vi "ttm_aecontrol_poller.vi"() -> ()   [LabVIEW 2011]
doc: "This is the sample data playback waveform and data logging example program. Sample data points are generated using MX Sample Data Array Generator.vi. You will need to replace this VI with your own code. New sample data is sent to the controller each time a status message is recieved from the controller that the next random buffer is running.\nThis program also shows you how to use Active X events. These are used to notify the program when a data buffer is ready for collection and when to load a new buffer of sample data points. Two separate event queues are used: one for data logging and the other for general status, such as when a sample data point buffer can be sent to the controller. Each event handler must run in parallel loops as execution passes to MX Handle Status Change Event.vi and MX Handle Data Ready Event.vi and will not come out of them until an event is received from the console program. When modifiying this example for your own use you may want to setup a third loop to be doing other processing, or you could add code to manipulate the data buffer in the data monitoring loop."
panel:
  out "Number of points":i32=1000
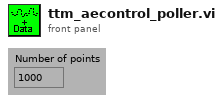
[diagram p1: front panel]
types:
  T1 = cluster{"Data Sample Format (0)":i8, "Loop code (2)":i8, "Target Amplitude (32767)":i16, "Playback rate":dbl, "Playback Scale":dbl[], "Envelope Ramp Rate":dbl, "Filter Order (0)":i8, "Filter Type (0)":i8, "Filter Bandwidth":dbl}
  T2 = cluster{"Name":string, "Type":i32, "SI Full Scale":dbl, "Full Scale":dbl, "Units String":string, "Display Format":string, "Gauge Length":dbl}[][]
  T3 = cluster{"Device ID":i32, "Device Name":string, "Device Type":i32}[]
  T4 = cluster{"Axis Information Out[0]":cluster{"Device ID":i32, "Device Name":string, "Device Type":i32}, "Axis Information Out[1]":cluster{"Device ID":i32, "Device Name":string, "Device Type":i32}, "Axis Information Out[2]":cluster{"Device ID":i32, "Device Name":string, "Device Type":i32}, "Axis Information Out[3]":cluster{"Device ID":i32, "Device Name":string, "Device Type":i32}, "Axis Information Out[4]":cluster{"Device ID":i32, "Device Name":string, "Device Type":i32}, "Axis Information Out[5]":cluster{"Device ID":i32, "Device Name":string, "Device Type":i32}, "Axis Information Out[6]":cluster{"Device ID":i32, "Device Name":string, "Device Type":i32}, "Axis Information Out[7]":cluster{"Device ID":i32, "Device Name":string, "Device Type":i32}, "Axis Information Out[8]":cluster{"Device ID":i32, "Device Name":string, "Device Type":i32}}
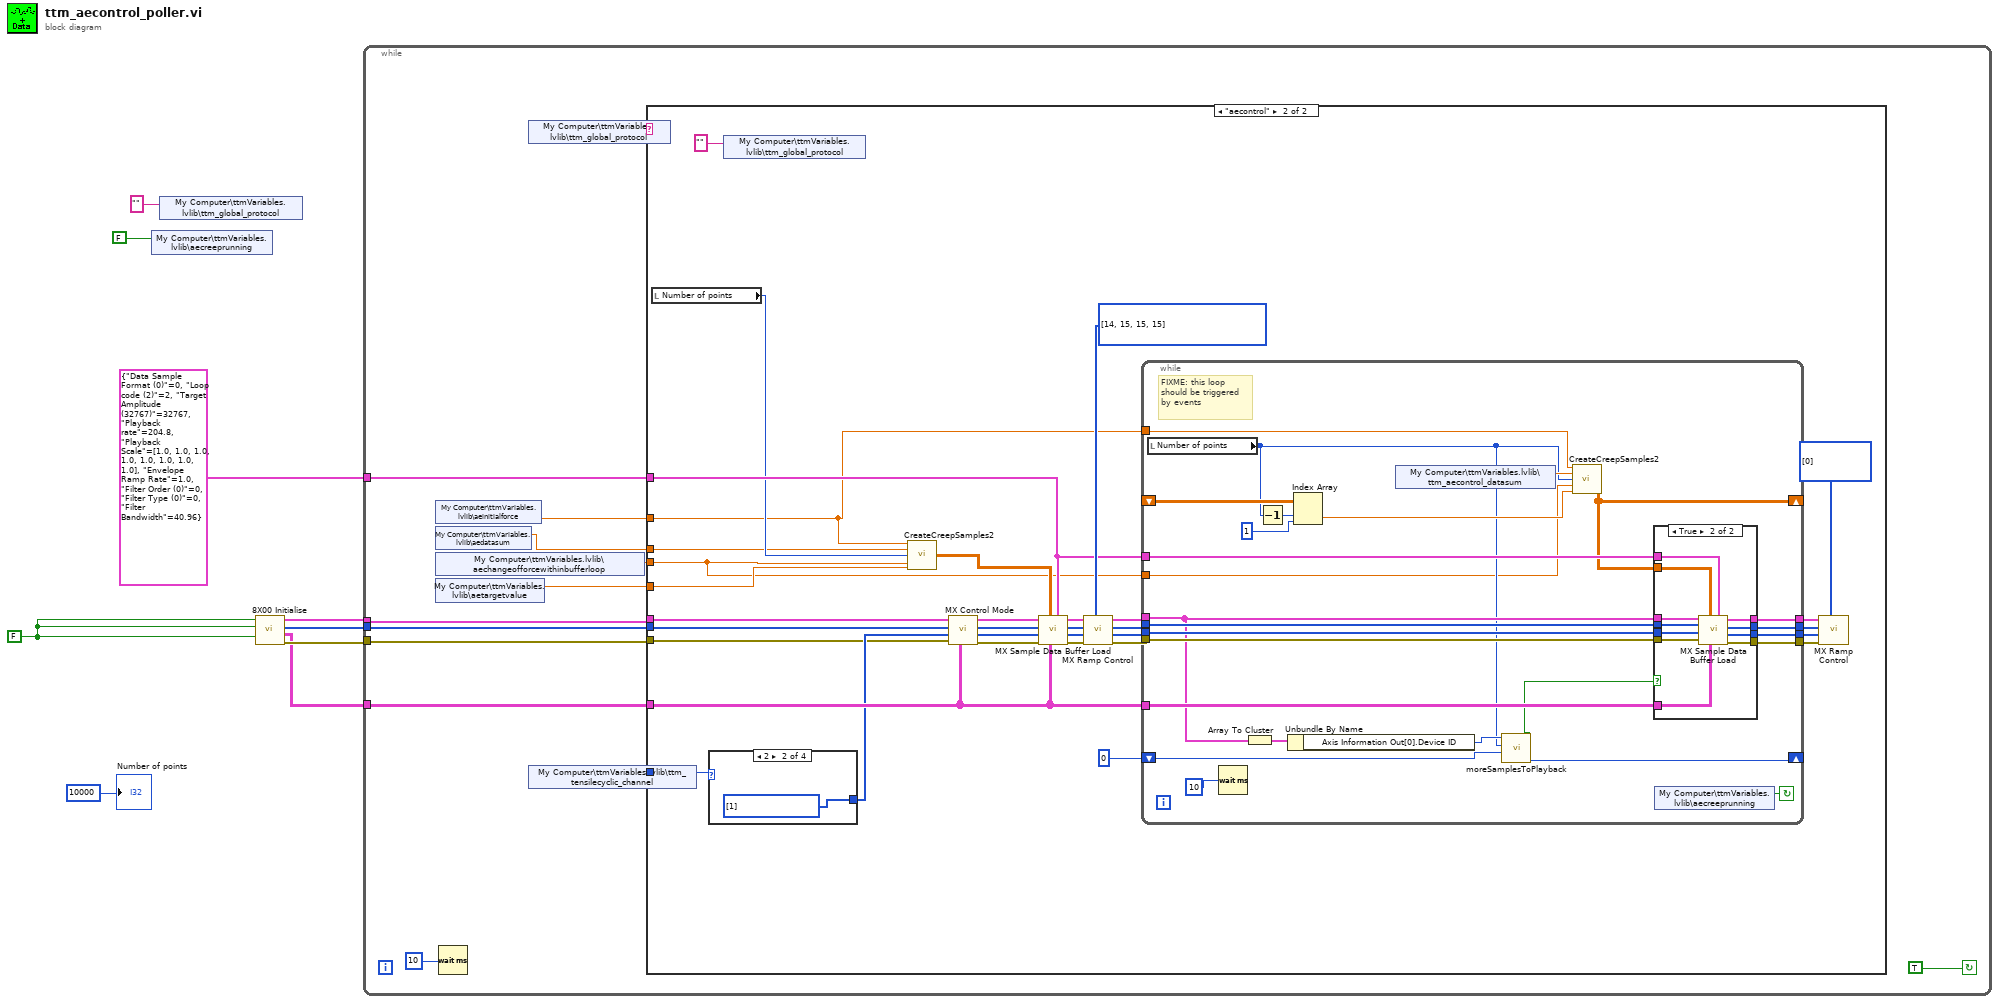
[diagram p0: block diagram]
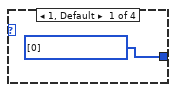
[diagram p3: hidden frame]
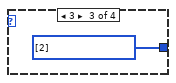
[diagram p4: hidden frame]
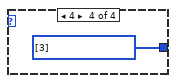
[diagram p5: hidden frame]
diagram:
  w6 = FALSE ("Reset")
  n1 = shared-variable "My Computer\\ttmVariables.lvlib\\aecreeprunning"(FALSE ("startCreep")) -> ()  [unwired: 1 in, 1 out]
  n2 = shared-variable "My Computer\\ttmVariables.lvlib\\ttm_global_protocol"("" ("protocol")) -> ()  [unwired: 1 in, 1 out]
  n3 = call "8X00 Initialise.vi"("Reset?"=w6, "Create DVM? (T)"=w6, "Create Console? (T)"=w6) -> ("error out"=w9:errorcluster, "Channel Data"=w8:T2, "Axis Selector"=w5:i32[], "Axis Information"=w7:T3)  [unwired: 1 in]
  n4 = while {
    tunnel: w8 -> [w22]
    tunnel: w7 -> [w18]
    tunnel: w9 -> [w16]
    tunnel: w5 -> [w17]
    tunnel: T1 {"Data Sample Format (0)"=0, "Loop code (2)"=2, "Target Amplitude (32767)"=32767, "Playback rate"=204.8, "Playback Scale"=[1.0, 1.0, 1.0, 1.0, 1.0, 1.0, 1.0, 1.0], "Envelope Ramp Rate"=1.0, "Filter Order (0)"=0, "Filter Type (0)"=0, "Filter Bandwidth"=40.96} ("Sample Data Playback Definition") -> [w14]
    stop <- TRUE continue-if-true
    n5 = shared-variable "My Computer\\ttmVariables.lvlib\\aeinitialforce"() -> (w12:dbl)  [unwired: 1 in, 1 out]
    n6 = shared-variable "My Computer\\ttmVariables.lvlib\\aedatasum"() -> (w13:dbl)  [unwired: 1 in, 1 out]
    n7 = shared-variable "My Computer\\ttmVariables.lvlib\\aechangeofforcewithinbufferloop"() -> (w11:dbl)  [unwired: 1 in, 1 out]
    n8 = shared-variable "My Computer\\ttmVariables.lvlib\\aetargetvalue"() -> (w19:dbl)  [unwired: 1 in, 1 out]
    n9 = Wait (ms)(milliseconds to wait=u32 10) -> ()  [unwired: 1 out]
    n10 = shared-variable "My Computer\\ttmVariables.lvlib\\ttm_global_protocol"() -> (w10:string)  [unwired: 1 in, 1 out]
    n11 = shared-variable "My Computer\\ttmVariables.lvlib\\ttm_tensilecyclic_channel"() -> (w15:i32)  [unwired: 1 in, 1 out]
    n12 = case shown="\"aecontrol\"" w10 {
      tunnel: w22 -> [_ w40]
      tunnel: w19 -> [_ w28]
      tunnel: w18 -> [_ w35]
      tunnel: w17 -> [_ w34]
      tunnel: w16 -> [_ w32]
      tunnel: w15 -> [_ w46]
      tunnel: w14 -> [_ w31]
      tunnel: w13 -> [_ w27]
      tunnel: w12 -> [_ w25]
      tunnel: w11 -> [_ w24]
      frame "False", Default {
      }
      frame "aecontrol" {
        w41 = u16[] [0] items=["Stop", "Start or continue", "Hold", "Continue", "Return ramp to set level at fixed rate", "Reserved", "Reserved", "Start Random without demand hold", "Start Random with demand hold", "Prepare Random Start without demand hold", "Prepare Random Start with demand hold", "Unslave", "Reserved", "Reserved", "Start Sample Data Playback or Resume", "Prepare for Start of Sample Data", "Reserved", "Reserved", "Resume Playback", "Start an electromechanical frame return"] ("Ramp Control")
        w51 = u16[] [14, 15, 15, 15] items=["Stop", "Start or continue", "Hold", "Continue", "Return ramp to set level at fixed rate", "Reserved", "Reserved", "Start Random without demand hold", "Start Random with demand hold", "Prepare Random Start without demand hold", "Prepare Random Start with demand hold", "Unslave", "Reserved", "Reserved", "Start Sample Data Playback or Resume", "Prepare for Start of Sample Data", "Reserved", "Reserved", "Resume Playback"] ("Ramp Control")
        n13 = local read "Number of points"() -> (w29:i32)
        n14 = case shown="2" w46 {
          tunnel: [w56 w57 w58 w59] -> w33
          frame 1, Default {
            w56 = u16[] [0] items=["Channel 1", "Channel 2", "Channel 3", "Channel 4"] ("Choose channel to apply\nthe setpoint")
          }
          frame 2 {
            w57 = u16[] [1] items=["Channel 1", "Channel 2", "Channel 3", "Channel 4"] ("Choose channel to apply\nthe setpoint")
          }
          frame 3 {
            w58 = u16[] [2] items=["Channel 1", "Channel 2", "Channel 3", "Channel 4"] ("Choose channel to apply\nthe setpoint")
          }
          frame 4 {
            w59 = u16[] [3] items=["Channel 1", "Channel 2", "Channel 3", "Channel 4"] ("Choose channel to apply\nthe setpoint")
          }
        }
        n15 = shared-variable "My Computer\\ttmVariables.lvlib\\ttm_global_protocol"("" ("protocol")) -> ()  [unwired: 1 in, 1 out]
        n16 = call "CreateCreepSamples2.vi"("setValueForAESum"=w25, "AEdataSum"=w27, "outputLength"=w29, "changeOfForceWithinBufferLoop"=w24, "initialOrPreviousForce"=w28) -> ("output array"=w30:dbl[][])  [unwired: 10 in]
        n17 = call "MX Control Mode.vi"("Channel Data"=w40, "error in (no error)"=w32, "Control Modes"=w33, "Axis Selector"=w34, "Axis Information"=w35) -> ("error out"=w36:errorcluster, "Control Modes out"=w37:u16[], "Axis Selector out"=w38:i32[], "Axis Information out"=w39:T3)  [unwired: 1 in]
        n18 = call "MX Sample Data Buffer Load.vi"("Sample Data Playback Definition"=w31, "Channel Data"=w40, "Sample Data"=w30, "error in (no error)"=w36, "Channels In"=w37, "Axis Selector In"=w38, "Axis Information In"=w39) -> ("error out"=w53:errorcluster, "Channels Out"=w52:u16[], "Axis Selector Out"=w54:i32[], "Axis Information Out"=w55:T3)  [unwired: 1 in]
        n19 = call "MX Ramp Control.vi"("Ramp Control"=w51, "error in (no error)"=w53, "Channels In"=w52, "Axis Selector In"=w54, "Axis Information In"=w55) -> ("error out"=w48:errorcluster, "Channels Out"=w50:u16[], "Axis Selector Out"=w49:i32[], "Axis Information Out"=w47:T3)  [unwired: 2 in]
        n20 = while {
          tunnel: w47 -> [w74]
          tunnel: w49 -> [w85]
          tunnel: w50 -> [w78]
          tunnel: w48 -> [w84]
          tunnel: [w75] -> w45
          tunnel: [w83] -> w44
          tunnel: [w82] -> w43
          tunnel: [w81] -> w42
          tunnel: w31 -> [w73]
          tunnel: w40 -> [w80]
          shift-right: [w69] -> _
          shift-left: _ -> [w72]
          shift-right: [w63] -> _
          shift-left: 0 -> [w62]
          tunnel: w25 -> [w61]
          tunnel: w24 -> [w60]
          stop <- w79 continue-if-true
          # "FIXME: this loop \nshould be triggered \nby events"
          n21 = local read "Number of points"() -> (w64:i32)
          n22 = Wait (ms)(milliseconds to wait=u32 10) -> ()  [unwired: 1 out]
          n23 = Array To Cluster(array=w74) -> (cluster=w76:T4)
          n24 = Decrement(x=w64) -> (x-1=w70:i32)
          n25 = Unbundle By Name(w76) -> ("Axis Information Out[0].Device ID"=w65:i32)
          n26 = Index Array(array=w72, index (row)=w70, index (col)=1) -> (element=w68:dbl)
          n27 = shared-variable "My Computer\\ttmVariables.lvlib\\ttm_aecontrol_datasum"() -> (w67:dbl)  [unwired: 1 in, 1 out]
          n28 = call "moreSamplesToPlayback.vi"("Device"=w65, "playbackCycleLength"=w64, "previousSampleCycle"=w62) -> ("ReadyForMore"=w66:bool, "currentSampleCycle"=w63:i32)  [unwired: 6 in]
          n29 = call "CreateCreepSamples2.vi"("setValueForAESum"=w61, "AEdataSum"=w67, "outputLength"=w64, "changeOfForceWithinBufferLoop"=w60, "initialOrPreviousForce"=w68) -> ("output array"=w69:dbl[][])  [unwired: 10 in]
          n30 = case shown="True" w66 {
            tunnel: w85 -> [w88 w100]
            tunnel: w84 -> [w86 w99]
            tunnel: [w88 w98] -> w83
            tunnel: [w87 w97] -> w82
            tunnel: [w86 w96] -> w81
            tunnel: w73 -> [_ w95]
            tunnel: w80 -> [_ w94]
            tunnel: w69 -> [_ w93]
            tunnel: w78 -> [w87 w92]
            tunnel: [w89 w91] -> w75
            tunnel: w74 -> [w89 w90]
            frame False {
            }
            frame True {
              n31 = call "MX Sample Data Buffer Load.vi"("Sample Data Playback Definition"=w95, "Channel Data"=w94, "Sample Data"=w93, "error in (no error)"=w99, "Channels In"=w92, "Axis Selector In"=w100, "Axis Information In"=w90) -> ("error out"=w96:errorcluster, "Channels Out"=w97:u16[], "Axis Selector Out"=w98:i32[], "Axis Information Out"=w91:T3)  [unwired: 1 in]
            }
          }
          n32 = shared-variable "My Computer\\ttmVariables.lvlib\\aecreeprunning"() -> (w79:bool)  [unwired: 1 in, 1 out]
        }
        n33 = call "MX Ramp Control.vi"("Ramp Control"=w41, "error in (no error)"=w42, "Channels In"=w43, "Axis Selector In"=w44, "Axis Information In"=w45) -> ()  [unwired: 2 in, 4 out]
      }
    }
  }
  "Number of points" <- 10000 ("Number of points")
